vi "NMRglobal2.vi"() -> ()   [LabVIEW 2013]
uses:
  <vilib>/Analysis/2dsp.llb/Power Spectrum (DBL).vi
  <vilib>/Analysis/NI_AALBase.lvlib
  <vilib>/Analysis/NI_AALPro.lvlib
panel:
  out "FFT Vrms":dbl[](graph)
  out "NMR Ave Graph":cluster{dbl, "Step Width (MHz)":dbl, dbl[][]}(graph)
  in  "COM Port #":refnum<visa-resource-name>="COM9"
  in  "GPIB Addr (28)":refnum<visa-resource-name>="GPIB0::28::INSTR"
  out "Pedestal (V)":dbl=0.021996041666666424 format="%_2g"
  in  "Open Global Panel":bool=TRUE
  out "Peak center (MHz)":sgl=213.36272 format="%.3f"
  out "Telnet error out":errorcluster
  out "+3V supply":dbl=3.294 format="%_4g"
  out "Temp (C)":dbl=27.62 format="%_4g"
  out "RF OK":bool=TRUE
  out "Peak area (V-MHz)":sgl=0.0010715195 format="%.5f"
  out "NMR Graph + Fit":cluster{cluster{dbl, "Numeric":dbl}[]}[](graph)=[{[{213.31, "Numeric"=0.006518283333333701}, {213.311, "Numeric"=0.003388283333334973}, {213.312, "Numeric"=0.0009528833333361936}, {213.313, "Numeric"=0.0007120833333300741}, {213.314, "Numeric"=-0.0009341166666686496}, {213.315, "Numeric"=0.00021428333333256555}, {213.316, "Numeric"=-0.00044271666666625964}, {213.317, "Numeric"=-0.0017051166666651463}, {213.318, "Numeric"=-0.0044729166666640785}, {213.319, "Numeric"=-0.0014461166666694322}, {213.32, "Numeric"=-0.001224716666668315}, {213.321, "Numeric"=0.0009912833333327493}, {213.322, "Numeric"=-0.002398116666666235}, {213.323, "Numeric"=-0.002492916666665273}, {213.324, "Numeric"=-0.004093116666664363}, {213.325, "Numeric"=-0.002098716666668953}, {213.326, "Numeric"=-0.004009716666667992}, {213.327, "Numeric"=-0.0018261166666670853}, {213.328, "Numeric"=-0.0009479166666662257}, {213.329, "Numeric"=-0.002075116666665419}, {213.33, "Numeric"=-0.0023077166666646623}, {213.331, "Numeric"=0.0007542833333315097}, {213.332, "Numeric"=0.0005108833333323168}, {213.333, "Numeric"=0.0012620833333330667}, {213.334, "Numeric"=0.002207883333333771}, {213.335, "Numeric"=0.006048283333334421}, {213.336, "Numeric"=0.004783283333335022}, {213.337, "Numeric"=0.0049128833333319626}, {213.338, "Numeric"=0.0066370833333326065}, {213.339, "Numeric"=0.006255883333333205}, {213.34, "Numeric"=0.006469283333333752}, {213.341, "Numeric"=0.008977283333334245}, {213.342, "Numeric"=0.00737988333333469}, {213.343, "Numeric"=0.009677083333332392}, {213.344, "Numeric"=0.007968883333332889}, {213.345, "Numeric"=0.012955283333333331}, {213.346, "Numeric"=0.014136283333333721}, {213.347, "Numeric"=0.01641188333333405}, {213.348, "Numeric"=0.016682083333334347}, {213.349, "Numeric"=0.016446883333332815}, {213.35, "Numeric"=0.01920628333333315}, {213.351, "Numeric"=0.022060283333333437}, {213.352, "Numeric"=0.023708883333333673}, {213.353, "Numeric"=0.025952083333333847}, {213.354, "Numeric"=0.02438988333333398}, {213.355, "Numeric"=0.026322283333333217}, {213.356, "Numeric"=0.030649283333333395}, {213.357, "Numeric"=0.034570883333333524}, {213.358, "Numeric"=0.0379870833333336}, {213.359, "Numeric"=0.03589788333333363}, {213.36, "Numeric"=0.036403283333333605}, {213.361, "Numeric"=0.03840328333333361}, {213.362, "Numeric"=0.046297883333333636}, {213.363, "Numeric"=0.044387083333333605}, {213.364, "Numeric"=0.04607088333333352}, {213.365, "Numeric"=0.04394928333333341}, {213.36599999999999, "Numeric"=0.043122283333333206}, {213.367, "Numeric"=0.04108988333333399}, {213.368, "Numeric"=0.03605208333333385}, {213.369, "Numeric"=0.03400888333333367}, {213.37, "Numeric"=0.03626028333333344}, {213.371, "Numeric"=0.03240628333333315}, {213.37199999999999, "Numeric"=0.03084688333333281}, {213.373, "Numeric"=0.025182083333334347}, {213.374, "Numeric"=0.023111883333334055}, {213.375, "Numeric"=0.02373628333333372}, {213.376, "Numeric"=0.015455283333333333}, {213.377, "Numeric"=0.013268883333332884}, {213.378, "Numeric"=0.014877083333332389}, {213.379, "Numeric"=0.01077988333333469}, {213.38, "Numeric"=0.008477283333334244}, {213.381, "Numeric"=0.006569283333333752}, {213.382, "Numeric"=0.0008558833333332065}, {213.383, "Numeric"=0.002237083333332609}, {213.384, "Numeric"=0.0009128833333319625}, {213.385, "Numeric"=-0.0013167166666649792}, {213.386, "Numeric"=-0.001151716666665581}, {213.387, "Numeric"=-0.005292116666666232}, {213.388, "Numeric"=-0.003537916666666932}, {213.389, "Numeric"=-0.002589116666667682}, {213.39, "Numeric"=-0.0020457166666684873}, {213.391, "Numeric"=-0.004107716666664665}, {213.392, "Numeric"=-0.0005751166666654178}, {213.393, "Numeric"=0.00035208333333377334}, {213.394, "Numeric"=-0.004426116666667083}, {213.395, "Numeric"=-0.0036097166666679906}, {213.396, "Numeric"=-0.003498716666668955}, {213.397, "Numeric"=-0.0004931166666643644}, {213.398, "Numeric"=-0.0006929166666652734}, {213.399, "Numeric"=-0.002398116666666235}, {213.4, "Numeric"=-0.0006087166666672479}, {213.401, "Numeric"=-0.0013247166666683144}, {213.402, "Numeric"=0.0014538833333305676}, {213.403, "Numeric"=-0.0009729166666640789}, {213.404, "Numeric"=-0.0007051166666651454}, {213.405, "Numeric"=-4.271666666625859e-05}, {213.406, "Numeric"=0.003114283333332569}, {213.407, "Numeric"=-0.0003341166666686532}, {213.408, "Numeric"=0.0024120833333300742}, {213.409, "Numeric"=0.004252883333336191}, {213.41, "Numeric"=0.0038882833333349735}]}]
  out "# Good Spectra":i32=200
  out "Pedestal OK":bool=TRUE
  out "Sweep #":i32=4
  out "1st Sweep":bool
  out "ADC volts OK":bool=TRUE
  out "Peak Height Distribution":cluster{"Y":dbl[], "Y":dbl[]}[](graph)=[{"Y"=[0.008346695000000091, 0.008617285000000093, 0.008887875000000092, 0.009158465000000093, 0.009429055000000094, 0.009699645000000093, 0.009970235000000095, 0.010240825000000096, 0.010511415000000095, 0.010782005000000096, 0.011052595000000097, 0.011323185000000097, 0.011593775000000098, 0.011864365000000099, 0.012134955000000098, 0.0124055450000001, 0.0126761350000001, 0.0129467250000001, 0.013217315000000101, 0.013487905000000102, 0.013758495000000101, 0.014029085000000103, 0.014299675000000104, 0.014570265000000103, 0.014840855000000104, 0.015111445000000105, 0.015382035000000106, 0.015652625000000107, 0.015923215000000105, 0.016193805000000106, 0.016464395000000107, 0.01673498500000011, 0.01700557500000011, 0.01727616500000011, 0.017546755000000108, 0.01781734500000011, 0.01808793500000011, 0.01835852500000011, 0.018629115000000113, 0.018899705000000114, 0.019170295000000115, 0.019440885000000113, 0.019711475000000114, 0.019982065000000115, 0.020252655000000116, 0.020523245000000117, 0.020793835000000118, 0.021064425000000116, 0.021335015000000117, 0.021605605000000118, 0.02187619500000012, 0.02214678500000012, 0.02241737500000012, 0.02268796500000012, 0.02295855500000012, 0.02322914500000012, 0.023499735000000122, 0.023770325000000123, 0.024040915000000124, 0.024311505000000122, 0.024582095000000123, 0.024852685000000124, 0.025123275000000125, 0.025393865000000126, 0.025664455000000128, 0.02593504500000013, 0.026205635000000126, 0.026476225000000127, 0.02674681500000013, 0.02701740500000013, 0.02728799500000013, 0.027558585000000132, 0.02782917500000013, 0.02809976500000013, 0.02837035500000013, 0.028640945000000133, 0.028911535000000134, 0.029182125000000135, 0.029452715000000133, 0.029723305000000134, 0.029993895000000135, 0.030264485000000136, 0.030535075000000137, 0.030805665000000138, 0.031076255000000136, 0.03134684500000014, 0.03161743500000014, 0.03188802500000014, 0.03215861500000014, 0.03242920500000014, 0.03269979500000014, 0.032970385000000144, 0.033240975000000145, 0.033511565000000146, 0.03378215500000014, 0.03405274500000014, 0.03432333500000014, 0.03459392500000014, 0.034864515000000144, 0.035135105000000146], "Y"=[1.0, 0.0, 0.0, 0.0, 0.0, 0.0, 0.0, 0.0, 0.0, 0.0, 0.0, 0.0, 2.0, 0.0, 0.0, 2.0, 2.0, 0.0, 1.0, 3.0, 0.0, 1.0, 3.0, 1.0, 3.0, 3.0, 1.0, 3.0, 3.0, 3.0, 3.0, 1.0, 2.0, 2.0, 1.0, 6.0, 6.0, 3.0, 3.0, 1.0, 6.0, 4.0, 3.0, 1.0, 3.0, 7.0, 4.0, 2.0, 3.0, 4.0, 8.0, 6.0, 3.0, 3.0, 4.0, 4.0, 4.0, 6.0, 4.0, 5.0, 0.0, 4.0, 4.0, 3.0, 1.0, 3.0, 3.0, 3.0, 1.0, 1.0, 0.0, 0.0, 4.0, 5.0, 1.0, 2.0, 4.0, 2.0, 2.0, 0.0, 5.0, 0.0, 2.0, 2.0, 0.0, 0.0, 1.0, 1.0, 0.0, 0.0, 0.0, 1.0, 0.0, 0.0, 0.0, 0.0, 0.0, 0.0, 0.0, 1.0]}]
  out "S/N":dbl=4.324476074402461 format="%_3g"
  out "Peak mean (V)":dbl=0.02176165200000014 format="%_4g"
  out "Pedestal Diff (V)":sgl=-0.0009116333 format="%.3f"
  out "Peak amp (V)":sgl=0.04629788 format="%.3f"
  out "SMT error out":errorcluster
  out "Sample RMS (V)":dbl=0.001899009900990099 format="%.4f"
  in  "Sweep Mode":u16(ring)=3 items=["Off", "Single", "Auto", "Step"]
  # "E1039 NMR Panel"
  # "Results"
  # "A\nv\ne\nr\na\ng\ne"
  # "S\nw\ne\ne\np"
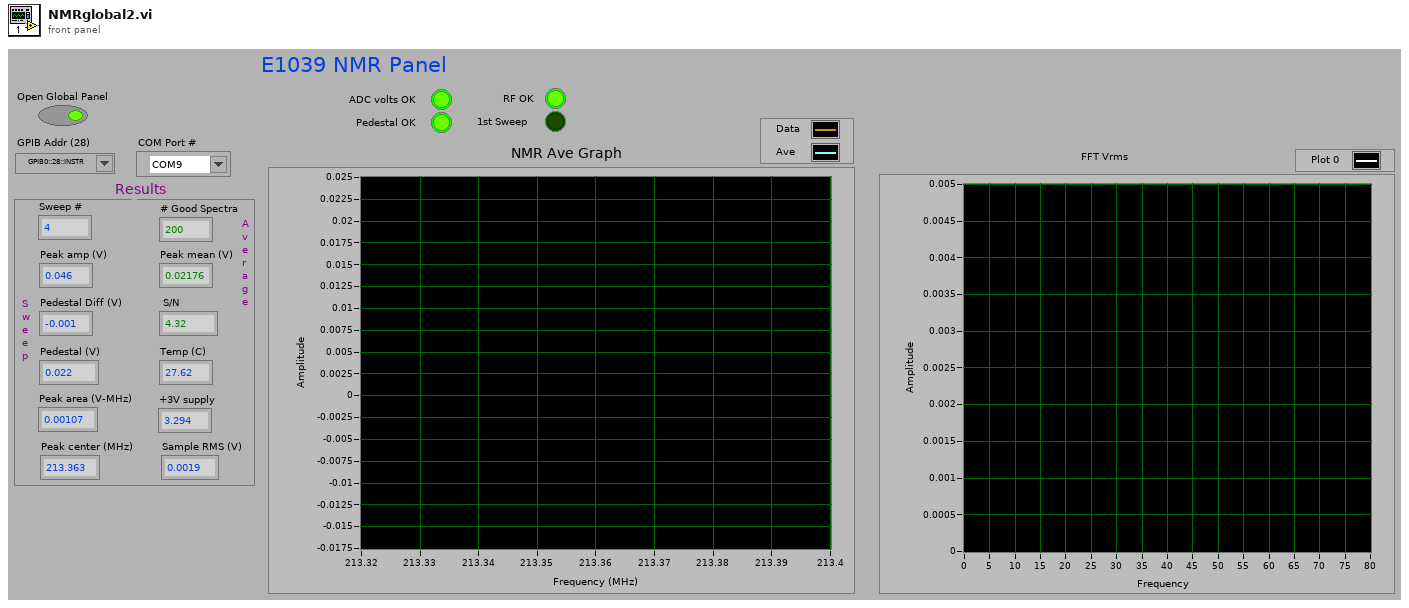
[diagram p1: front panel]
types:
  T1 = enum32{"Invalid", "Standard", "Closed", "Hidden", "Minimized", "Maximized"}
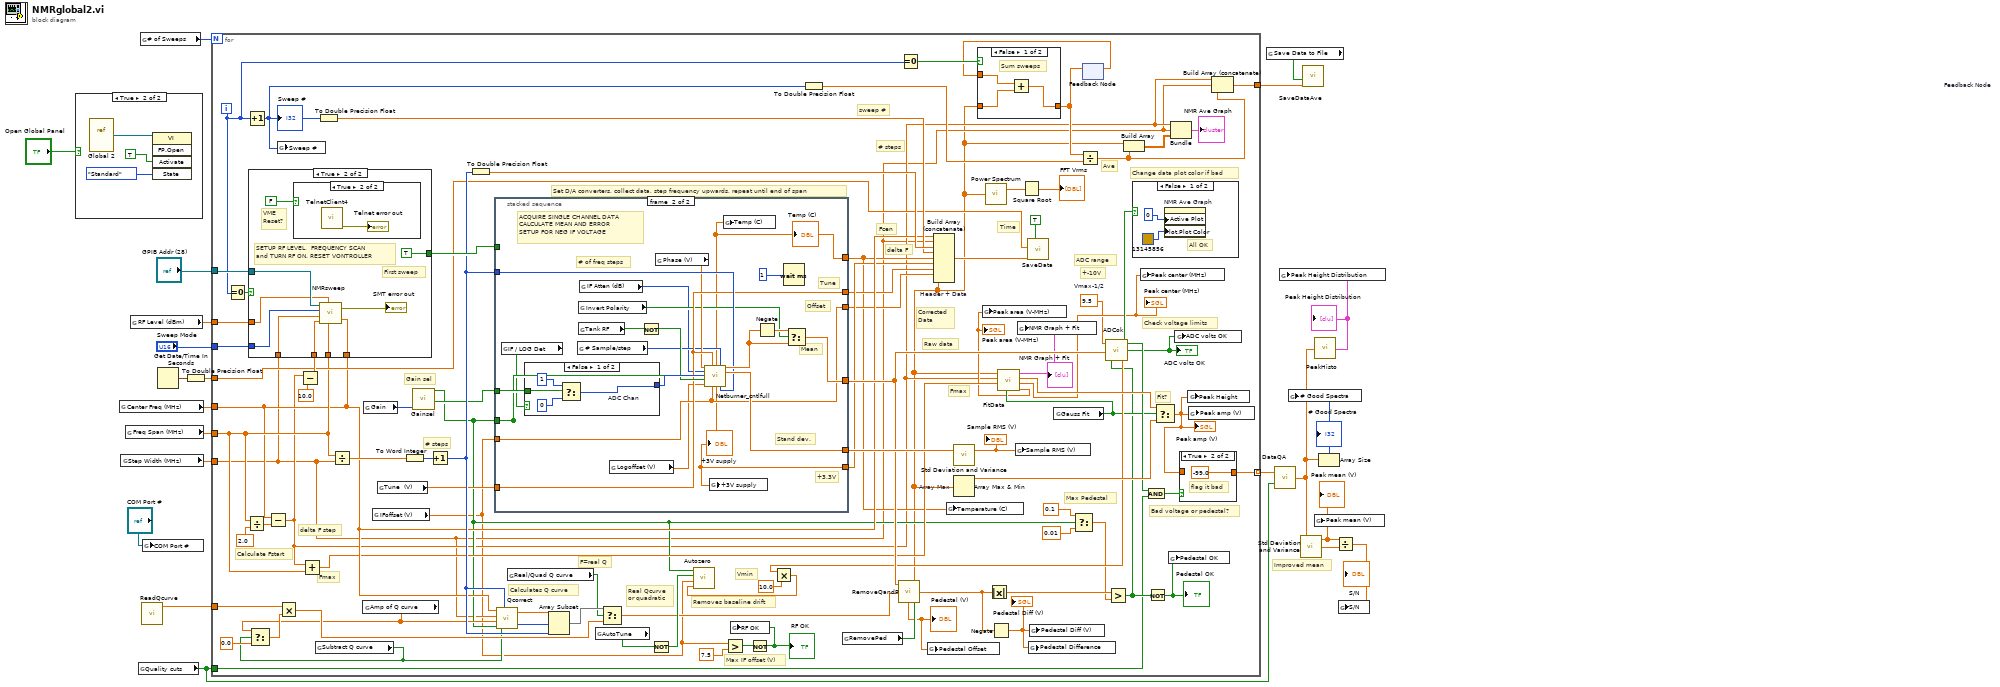
[diagram p0: block diagram]
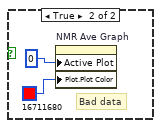
[diagram p4: hidden frame]
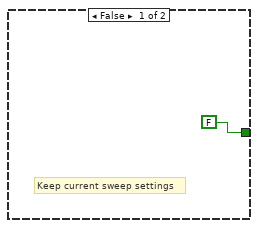
[diagram p6: hidden frame]
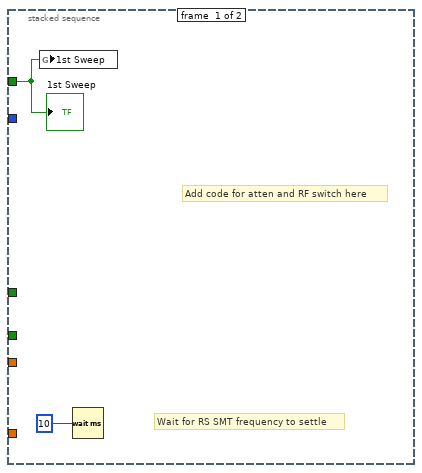
[diagram p8: hidden frame]
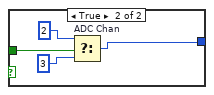
[diagram p9: hidden frame]
diagram:
  # "Improved mean"
  n1 = case shown="True" "Open Global Panel" {
    frame False {
    }
    frame True {
      n2 = vi-ref "Global 2.vi"() -> (w25:refnum<vi>)
      n3 = invoke class="VI" method="FP.Open"(reference=w25, "Activate"=TRUE, "State"=T1."Standard") -> ()  [unwired: 2 in, 5 out]
    }
  }
  n4 = global read "Global 2.vi" "Center Freq (MHz)"() -> (w15:dbl)
  n5 = global read "Global 2.vi" "Step Width (MHz)"() -> (w13:dbl)
  n6 = global read "Global 2.vi" "Freq Span (MHz)"() -> (w14:dbl)
  n7 = global read "Global 2.vi" "RF Level (dBm)"() -> (w16:dbl)
  n8 = global read "Global 2.vi" "Quality cuts"() -> (w12:bool)
  n9 = global read "Global 2.vi" "# of Sweeps"() -> (w17:i32)
  n10 = call "ReadQcurve.vi"() -> ("Array"=w1:dbl[])  [unwired: 2 in]
  n11 = global write "Global 2.vi" "COM Port #"("COM Port #") -> ()
  n12 = Get Date/Time In Seconds() -> (seconds since 1Jan1904=w19:timestamp)
  n13 = To Double Precision Float(number=w19) -> (double precision float=w2:dbl)
  n14 = for {
    N: w17 -> [_]
    tunnel: [w103] -> w22 mode=indexing
    tunnel: w12 -> [w49]
    tunnel: w15 -> [w87]
    tunnel: w14 -> [w91]
    tunnel: w13 -> [w34]
    tunnel: "Sweep Mode" -> [w96]
    tunnel: "GPIB Addr (28)" -> [w95]
    tunnel: w16 -> [w94]
    tunnel: w2 -> [w92]
    tunnel: w1 -> [w80]
    tunnel: [w33] -> w4
    i -> [w29]
    w43 = 9.5  # Vmax-1/2
    # "Check voltage limits"
    # "Ave"
    # "Max Pedestal"
    # "Gain sel"
    # "F=real Q"
    # "Real Qcurve\nor quadratic"
    # "+-10V"
    # "Change data plot color if bad"
    # "Max IF offset (V)"
    # "Fmax"
    # "Fit?"
    # "Fmax"
    # "Time"
    # "Vmin"
    # "Raw data"
    # "Corrected\nData"
    # "Fcen"
    # "delta F"
    # "# steps"
    # "ADC range"
    # "sweep #"
    # "Set D/A converters, collect data, step frequency upwards, repeat until end of span"
    # "Calculates Q curve"
    # "Removes baseline drift"
    # "Bad voltage or pedestal?"
    # "# steps"
    # "Calculate Fstart"
    # "delta F step"
    n15 = Equal To 0?(x=w29) -> (x = 0?=w105:bool)
    n16 = Divide(x=w91, y=sgl 2.0) -> (x/y=w112:dbl)
    n17 = Increment(x=w29) -> (x+1=w47:i32)
    "Sweep #" <- w47
    n18 = Subtract(x=w87, y=w112) -> (x-y=w35:dbl)
    n19 = global write "Global 2.vi" "Sweep #"(w47) -> ()
    n20 = Subtract(x=w35, y=10.0) -> (x-y=w110:dbl)
    n21 = case shown="True" w105 {
      tunnel: w110 -> [_ w135]
      tunnel: w34 -> [_ w133]
      tunnel: w87 -> [_ w132]
      tunnel: w91 -> [_ w134]
      tunnel: [FALSE TRUE] -> w104
      tunnel: w96 -> [_ w129]
      tunnel: w95 -> [_ w128]
      tunnel: w94 -> [_ w127]
      frame False {
        # "Keep current sweep settings"
      }
      frame True {
        # "VME\nReset?"
        # "First sweep"
        # "SETUP RF LEVEL,  FREQUENCY SCAN\nand TURN RF ON. RESET VONTROLLER"
        n22 = case shown="True" FALSE {
          frame False {
          }
          frame True {
            n23 = call "TelnetClient4.vi"() -> ("Telnet error"=→"Telnet error out":errorcluster)  [unwired: 4 in, 3 out]
          }
        }
        n24 = call "NMRsweep.vi"("Center Freq (MHz)"=w132, "Freq Span (MHz)"=w134, "RF Level (dBm)"=w127, "Foffset (MHz)"=w135, "Step Width (MHz)"=w133, "Sweep Mode"=w129, "GPIB Addr (28)"=w128) -> ("error out"=→"SMT error out":errorcluster)
      }
    }
    n25 = Add(x=w35, y=w91) -> (x+y=w85:dbl)
    n26 = global read "Global 2.vi" "Subtract Q curve"() -> (w68:bool)
    n27 = To Double Precision Float(number=w47) -> (double precision float=w97:dbl)
    n28 = Divide(x=w91, y=w34) -> (x/y=w114:dbl)
    n29 = global read "Global 2.vi" "Amp of Q curve"() -> (w69:dbl)
    n30 = Select(t=w69, s=w68, f=0.0) -> (s? t:f=w77:dbl)
    n31 = Multiply(x=w80, y=w77) -> (x*y=w79:dbl[])
    n32 = global read "Global 2.vi" "Gain"() -> (w38:enum16{"LOW", "HI", "MAX"})
    n33 = global read "Global 2.vi" "IFoffset (V)"() -> (w32:dbl)
    n34 = global read "Global 2.vi" "Tune  (V)"() -> (w70:dbl)
    n35 = To Word Integer(number=w114) -> (16bit integer=w111:i16)
    n36 = call "Gainsel.vi"("Gain"=w38) -> ("LO"=w39:bool, "MAX"=w37:bool)  [unwired: 1 out]
    n37 = Increment(x=w111) -> (x+1=w99:i16)
    n38 = To Double Precision Float(number=w99) -> (double precision float=w98:dbl)
    n39 = stacked-sequence {
      tunnel: [_ w154] -> w107
      tunnel: [_ w158] -> w93
      tunnel: w99 -> [_ w152]
      tunnel: w32 -> [_ w149]
      tunnel: w39 -> [_ w156]
      tunnel: w104 -> [w137 _]
      tunnel: w70 -> [_ w150]
      tunnel: [_ w140] -> w54
      tunnel: [_ w139] -> w76
      tunnel: [_ w150] -> w75
      tunnel: [_ w149] -> w74
      tunnel: [_ w148] -> _
      tunnel: w37 -> [_ w148]
      frame #0 {
        # "Add code for atten and RF switch here"
        # "Wait for RS SMT frequency to settle"
        n40 = global write "Global 2.vi" "1st Sweep"(w137) -> ()
        n41 = Wait (ms)(milliseconds to wait=10) -> ()  [unwired: 1 out]
        "1st Sweep" <- w137
      }
      frame #1 {
        # "+3.3V"
        # "Offset"
        # "Tune"
        # "Stand dev."
        # "Mean"
        # "ACQUIRE SINGLE CHANNEL DATA\nCALCULATE MEAN AND ERROR\nSETUP FOR NEG IF VOLTAGE"
        # "# of freq steps"
        n42 = global read "Global 2.vi" "IF / LOG Det"() -> (w145:bool)
        n43 = case shown="False" w145 {
          tunnel: w156 -> [w163 w164]
          tunnel: [w160 w165] -> w153
          frame False {
            n44 = Select "ADC Chan"(t=1, s=w163, f=0) -> (s? t:f=w160:i32)
          }
          frame True {
            n45 = Select "ADC Chan"(t=2, s=w164, f=3) -> (s? t:f=w165:i32)
          }
        }
        n46 = global read "Global 2.vi" "# Sample/step"() -> (w142:i32)
        n47 = global read "Global 2.vi" "Tank RF"() -> (w144:bool)
        n48 = global read "Global 2.vi" "Invert Polarity"() -> (w143:bool)
        n49 = global read "Global 2.vi" "IF Atten (dB)"() -> (w141:i8)
        n50 = global read "Global 2.vi" "Logoffset (V)"() -> (w146:dbl)
        n51 = Not(x=w144) -> (.not. x?=w151:bool)
        n52 = global read "Global 2.vi" "Phase (V)"() -> (w147:dbl)
        n53 = call "Netburner_cntlfull.vi"("Phase Volt"=w147, "Tune Volt"=w150, "# Data"=w142, "IF Atten (dB)"=w141, "NMR ADC"=w153, "Hi Gain"=w148, "Tank RF"=w151, "LogOff Volt"=w146, "IFOff Volt"=w149, "# f steps"=w152) -> ("Temp (C)"=w140:dbl, "ADC value"=w155:dbl[], "ADC error"=w154:dbl[], "Volts"=w139:dbl)  [unwired: 2 out]
        "Temp (C)" <- w140
        "+3V supply" <- w139
        n54 = global write "Global 2.vi" "+3V supply"(w139) -> ()
        n55 = global write "Global 2.vi" "Temp (C)"(w140) -> ()
        n56 = Negate(x=w155) -> (-x=w157:dbl[])
        n57 = Wait (ms)(milliseconds to wait=1) -> ()  [unwired: 1 out]
        n58 = Select(t=w157, s=w143, f=w155) -> (s? t:f=w158:dbl[])
      }
    }
    n59 = call "Qcorrect.vi"("Subtract Q curve"=w68, "Nstep"=w99, "Max Gain"=w37, "Amp of Q curve"=w69, "Step Width (MHz)"=w34, "Center Freq (MHz)"=w87) -> ("Start"=w108:i32, "Array"=w109:dbl[])
    n60 = global read "Global 2.vi" "Real/Quad Q curve"() -> (w67:bool)
    n61 = Array Subset "Array Subset"(array=w109, index=w108, length=w99) -> (w82:dbl[])
    n62 = global read "Global 2.vi" "AutoTune"() -> (w65:bool)
    n63 = Select(t=w82, s=w67, f=w79) -> (s? t:f=w81:dbl[])
    n64 = Not(x=w65) -> (.not. x?=w83:bool)
    n65 = Greater?(x=w32, y=7.5) -> (0:w88:bool)
    n66 = Not(x=w88) -> (.not. x?=w61:bool)
    "RF OK" <- w61
    n67 = global write "Global 2.vi" "RF OK"(w61) -> ()
    n68 = To Double Precision Float(number=w47) -> (double precision float=w41:dbl)
    n69 = global read "Global 2.vi" "RemovePed"() -> (w66:bool)
    n70 = call "RemoveQandP.vi"("Subtract Ped?"=w66, "Qcurve"=w81, "Raw data"=w93) -> ("Ped L-R"=w100:dbl, "Corrected data"=w26:dbl[], "Ped Offfset"=w53:dbl)
    "Pedestal (V)" <- w53
    n71 = Equal To 0?(x=w29) -> (x = 0?=w46:bool)
    n72 = global write "Global 2.vi" "Pedestal Offset"(w53) -> ()
    n73 = Build Array (concatenate) "Header + Data"(w87, w34, w98, w97, w54, w76, w75, w74, w26) -> (w30:dbl[])
    n74 = global write "Global 2.vi" "Temperature (C)"(w54) -> ()
    n75 = call <vilib>:"Std Deviation and Variance.vi"("X"=w107) -> ("mean"=w59:dbl)  [unwired: 1 in, 2 out]
    "Sample RMS (V)" <- w59
    n76 = Array Max & Min "Array Max"(array=w26) -> (max value=w90:dbl)  [unwired: 3 out]
    n77 = call-poly <vilib>:"Power Spectrum.vi"("X"=w26) -> ("Power Spectrum"=w28:dbl[])  [unwired: 1 out]
    n78 = Absolute Value ("Abs Value")(x=w100) -> (abs(x)=w101:dbl)
    n79 = Negate(x=w100) -> (-x=w55:dbl)
    "Pedestal Diff (V)" <- w55
    n80 = global write "Global 2.vi" "Sample RMS (V)"(w59) -> ()
    n81 = Square Root(x=w28) -> (sqrt(x)=→"FFT Vrms":dbl[])
    n82 = call "SaveData.vi"("Array"=w30, "Save Data to File"=TRUE, "Ext time (sec)"=w92) -> ()  [unwired: 1 out]
    n83 = global write "Global 2.vi" "Pedestal Difference"(w55) -> ()
    n84 = global write "Global 2.vi" "Pedestal Diff (V)"(w55) -> ()
    n85 = global read "Global 2.vi" "Gauss Fit"() -> (w64:bool)
    n86 = call "FitData.vi"("Fit?"=w64, "Fmax"=w85, "Fmin"=w35, "Yarray"=w26) -> ("Peak Area (V-MHz)"=w60:dbl, "Center Freq (MHz)"=w58:dbl, "Amplitude (V)"=w86:dbl, "NMR Graph + Fit"=w56:cluster{cluster{dbl, "Numeric":dbl}[]}[])  [unwired: 1 out]
    "NMR Graph + Fit" <- w56
    "Peak area (V-MHz)" <- w60
    "Peak center (MHz)" <- w58
    n87 = global write "Global 2.vi" "Peak area (V-MHz)"(w60) -> ()
    n88 = global write "Global 2.vi" "NMR Graph + Fit"(w56) -> ()
    n89 = Select(t=0.1, s=w37, f=0.01) -> (s? t:f=w48:dbl)
    n90 = feedback #1 "Feedback Node"() -> (w45:dbl[])  [unwired: 1 in]
    n91 = case shown="False" w46 {
      tunnel: w26 -> [w116 w118]
      tunnel: [w115 w118] -> w42
      tunnel: w45 -> [w117 _]
      frame False {
        # "Sum sweeps"
        n92 = Add(x=w117, y=w116) -> (x+y=w115:dbl[])
      }
      frame True {
        # "Initialize"
      }
    }
    n93 = Divide(x=w42, y=w41) -> (x/y=w36:dbl[])
    n94 = feedback-in #1(w42) -> ()
    n95 = Greater?(x=w101, y=w48) -> (0:w50:bool)
    n96 = call "ADCok.vi"("PedOK"=w50, "Array"=w93, "Vmax-1/2"=w43) -> ("Vmin"=w73:dbl, "ADC voltages OK"=w63:bool, "Allok"=w84:bool)
    "ADC volts OK" <- w63
    n97 = Multiply(x=w73, y=10.0) -> (x*y=w71:dbl)
    n98 = call "Autozero.vi"("Vmin (V)"=w71, "IFoffset (V)"=w32, "Enable"=w83, "Max Gain"=w37) -> ()
    n99 = Build Array "Build Array"(w26, w36) -> (w40:dbl[][])
    n100 = case shown="False" w84 {
      frame False {
        # "All OK"
        n101 = property on="NMR Ave Graph" class="WFGraph (strict)"("Active Plot"=0, "Plot.Plot Color"=u32 13145856) -> ()  [unwired: 2 in, 2 out]
      }
      frame True {
        # "Bad data"
        n102 = property on="NMR Ave Graph" class="WFGraph (strict)"("Active Plot"=0, "Plot.Plot Color"=u32 16711680) -> ()  [unwired: 2 in, 2 out]
      }
    }
    n103 = global write "Global 2.vi" "Peak center (MHz)"(w58) -> ()
    n104 = And(x=w84, y=w49) -> (x .and. y?=w102:bool)
    n105 = Not(x=w50) -> (.not. x?=w62:bool)
    "Pedestal OK" <- w62
    n106 = Select(t=w86, s=w64, f=w90) -> (s? t:f=w57:dbl)
    "Peak amp (V)" <- w57
    n107 = global write "Global 2.vi" "Pedestal OK"(w62) -> ()
    n108 = Bundle(w35, "Step Width (MHz)"=w34, w40) -> (→"NMR Ave Graph":cluster{dbl, "Step Width (MHz)":dbl, dbl[][]})  [unwired: 1 in]
    n109 = global write "Global 2.vi" "ADC volts OK"(w63) -> ()
    n110 = case shown="True" w102 {
      tunnel: [w123 -99.0] -> w103
      tunnel: w57 -> [w123 _]
      frame False {
        # "Data OK"
      }
      frame True {
        # "flag it bad"
      }
    }
    n111 = global write "Global 2.vi" "Peak Height"(w57) -> ()
    n112 = global write "Global 2.vi" "Peak amp (V)"(w57) -> ()
    n113 = Build Array (concatenate) "Build Array"(w35, w34, w36) -> (w33:dbl[])
  }
  n114 = global read "Global 2.vi" "Save Data to File"() -> (w3:bool)
  n115 = call "DataQA.vi"("Quality cuts"=w12, "Data In"=w22) -> ("Data Out"=w21:dbl[])
  n116 = call <vilib>:"Std Deviation and Variance.vi"("X"=w21) -> ("mean"=w10:dbl, "standard deviation"=w18:dbl)  [unwired: 1 in, 1 out]
  "Peak mean (V)" <- w10
  n117 = call "SaveDataAve.vi"("Array"=w4, "Save Data to File"=w3) -> ()  [unwired: 1 in, 1 out]
  n118 = call "PeakHisto.vi"("Data Out"=w21) -> ("XY Graph"=w8:cluster{"Y":dbl[], "Y":dbl[]}[])
  "Peak Height Distribution" <- w8
  n119 = global write "Global 2.vi" "Peak Height Distribution"(w8) -> ()
  n120 = global write "Global 2.vi" "Peak mean (V)"(w10) -> ()
  n121 = Array Size(array=w21) -> (size(s)=w9:i32)
  "# Good Spectra" <- w9
  n122 = global write "Global 2.vi" "# Good Spectra"(w9) -> ()
  n123 = Divide(x=w10, y=w18) -> (x/y=w11:dbl)
  "S/N" <- w11
  n124 = global write "Global 2.vi" "S/N"(w11) -> ()
